vi "Launch File Actors.vi"(7 "error in":errorcluster, 10 "Controller in":refnum<class "Controller.lvclass">) -> (0 "error out":errorcluster, 3 "Controller out":refnum<class "Controller.lvclass">)   [LabVIEW 2014, in "Controller.lvlib" / "Controller.lvclass"]
uses:
  Controller.lvclass
  File Actor/File Actor.lvclass
  Messages/Saving File MSG/Save Main File MSG.lvclass
  Messages/Execute Write Main/Exe Write Main.lvclass
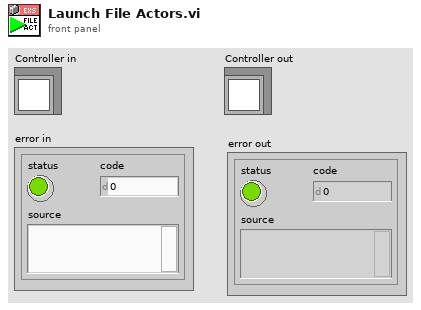
[diagram p1: front panel]
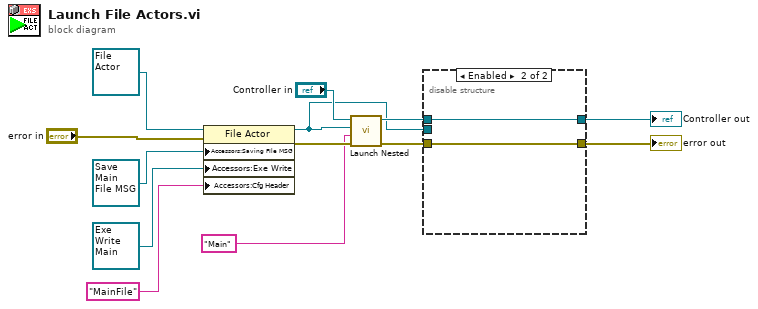
[diagram p0: block diagram]
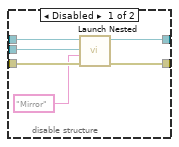
[diagram p2: hidden frame]
diagram:
  n1 = property class="File Actor"(reference=refnum<class "File Actor.lvclass"> refnum ("File Library.lvlib:File Actor"), error in="error in", "Accessors:Saving FIle MSG"=refnum<class "Save Main File MSG.lvclass"> refnum ("Controller.lvlib:Save Main File MSG"), "Accessors:Exe Write"=refnum<class "Exe Write Main.lvclass"> refnum ("Controller.lvlib:Exe Write Main"), "Accessors:Cfg Header"="MainFile" ("Cfg Header")) -> (reference out=w1:refnum<class "File Actor.lvclass">, error out=w7:errorcluster)
  n2 = call "Launch Nested.vi"("Error In"=w7, "ID"="Main", "Nested Actor"=w1, "Controller in"="Controller in") -> ("Error Out"=w2:errorcluster, "Controller out"=w6:refnum<class "Controller.lvclass">)  [unwired: 5 in, 1 out]
  n3 = disable-structure shown="Enabled" {
    disable-tunnel: w6 -> [w19 w21]
    disable-tunnel: [w18 w21] -> w5
    disable-tunnel: [w17 w20] -> w4
    disable-tunnel: w2 -> [w16 w20]
    disable-tunnel: w1 -> [w15 _]
    frame Disabled {
      n4 = call "Launch Nested.vi"("Error In"=w16, "ID"="Mirror", "Nested Actor"=w15, "Controller in"=w19) -> ("Error Out"=w17:errorcluster, "Controller out"=w18:refnum<class "Controller.lvclass">)  [unwired: 5 in, 1 out]
    }
    frame Enabled {
    }
  }
  "Controller out" <- w5
  "error out" <- w4
